vi "Status TimerList (Quick).vi"(8 "error in (no error)":errorcluster, 10 "Address (0)":i32, 11 "VISA resource name":refnum<visa-resource-name>) -> (0 "error out":errorcluster, 2 "Quick Timer":T1 {"Set-Time (s)" format="%<%H:%M>t"}, 3 "VISA resource name out":refnum<visa-resource-name>)   [LabVIEW 2016, in "Environment Chamber.lvlib" / "Climatic Chamber.lvlib"]
doc: "<b>Timer content monitor</b>\n\nReturns the settings of the Quick Timer."
uses:
  Climatic Chamber.lvlib
  Private/Type Defs/QuickTimer Cluster.ctl
  Private/Type Defs/Operation_Stop Mode Enum.ctl
  Private/Type Defs/TimerNumber Enum.ctl
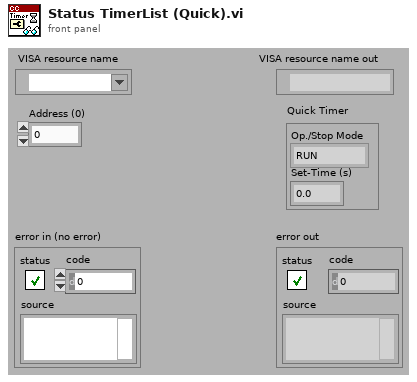
[diagram p1: front panel]
types:
  T1 = typedef "Environment Chamber.lvlib/Climatic Chamber.lvlib/QuickTimer Cluster.ctl" = cluster{"Op./Stop Mode":T2, "Set-Time (s)":dbl}
  T2 = typedef "Environment Chamber.lvlib/Climatic Chamber.lvlib/Operation_Stop Mode Enum.ctl" = enum16{"RUN", "CONSTANT", "STANDBY", "OFF"}
  T3 = typedef "Environment Chamber.lvlib/Climatic Chamber.lvlib/TimerNumber Enum.ctl" = enum16{"Quick Timer", "Start Timer", "End Timer"}
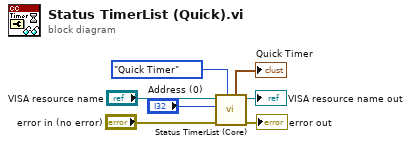
[diagram p0: block diagram]
diagram:
  n1 = call "Status TimerList (Core).vi"("Timer Number"=TimerNumber_Enum."Quick Timer", "error in (no error)"="error in (no error)", "Address (0)"="Address (0)", "VISA resource name"="VISA resource name") -> ("error out"=→"error out":errorcluster, "VISA resource name out"=→"VISA resource name out":refnum<visa-resource-name>, "Quick Timer"=→"Quick Timer":T1)  [unwired: 3 in, 2 out]
